vi "SizesofArray.vi"(11 "数组":u32[][](array[numeric])) -> (0 "NumCols_r":i32, 1 "NumRows_r":i32, 2 "NumCols":u32, 3 "NumRows":u32)   [LabVIEW 2014]
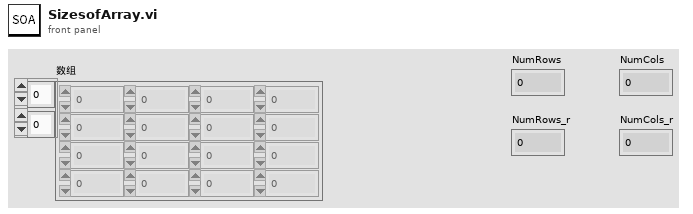
[diagram p1: front panel]
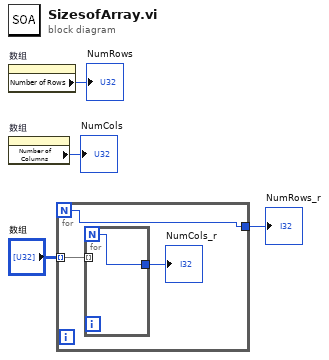
[diagram p0: block diagram]
diagram:
  n1 = property on="数组" class="Arr (严格)"() -> ("Number of Rows"=→"NumRows":u32)  [unwired: 2 in, 2 out]
  n2 = property on="数组" class="Arr (严格)"() -> ("Number of Columns"=→"NumCols":u32)  [unwired: 2 in, 2 out]
  n3 = for {
    N -> [w7]
    tunnel: "数组" -> [w6] mode=indexing
    tunnel: [w7] -> w2
    n4 = for {
      N -> [w8]
      tunnel: w6 -> [_] mode=indexing
      tunnel: [w8] -> w5
    }
    "NumCols_r" <- w5
  }
  "NumRows_r" <- w2
